vi "Set Project Path.vi"(0 "Project Path":path, 11 "error in (no error)":errorcluster) -> (15 "error out":errorcluster)   [LabVIEW 2021, in "Converter Reusables.lvlib"]
uses:
  Converter Reusables.lvlib
  controls/Dictionary States.ctl
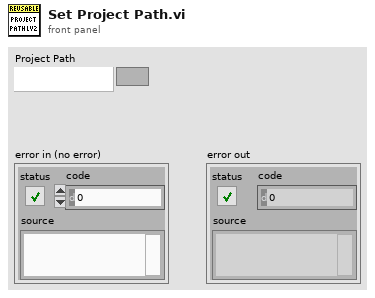
[diagram p1: front panel]
types:
  T1 = typedef "Converter Reusables.lvlib/Dictionary States.ctl" = enum16{"Set", "Get", "Delete", "Delete All"}
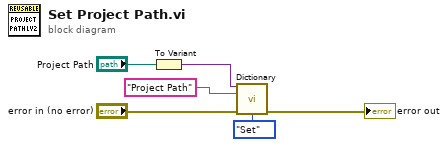
[diagram p0: block diagram]
diagram:
  n1 = To Variant(anything="Project Path") -> (Variant=w1:variant)
  n2 = call "Dictionary.vi"("Variant_In"=w1, "Key"="Project Path", "error in (no error)"="error in (no error)", "Dict States"=Dictionary_States."Set") -> ("error out"=→"error out":errorcluster)  [unwired: 10 in, 1 out]
